vi "Display Module - All Images Active.vi"(7 "Image Refs In":T1[](array[typedef])) -> (8 "Image Refs Out":T1[](array[typedef]))   [LabVIEW 2020]
uses:
  <vilib>/vision/Image Controls.llb/IMAQ Image.ctl
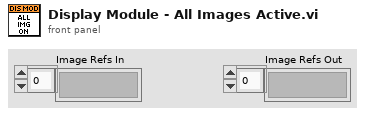
[diagram p1: front panel]
types:
  T1 = typedef "IMAQ Image.ctl" = refnum<image>
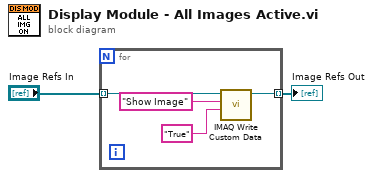
[diagram p0: block diagram]
diagram:
  n1 = for {
    tunnel: "Image Refs In" -> [w4] mode=indexing
    tunnel: [w3] -> w1 mode=indexing
    n2 = call "IMAQ Write Custom Data"("Custom Data In"="True", "Key"="Show Image", "Image"=w4) -> ("Image Out"=w3:T1)  [unwired: 7 in, 1 out]
  }
  "Image Refs Out" <- w1
